vi "TestVirtual6.vi"(0 "reference in":refnum<class "G#SubSubClass1.lvclass">, 5 "error in (no error)":errorcluster) -> (14 "reference out":refnum<class "G#SubSubClass1.lvclass">, 15 "MethodName":string[](array[string]), 19 "error out":errorcluster)   [LabVIEW 2010, in "G#SubSubClass1.lvclass"]
uses:
  G#SubSubClass1.lvclass
  G#SubClass1_class/G#SubClass1.lvclass
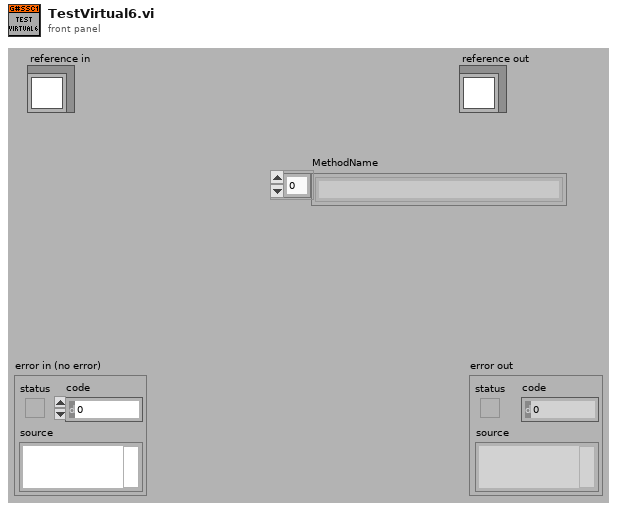
[diagram p1: front panel]
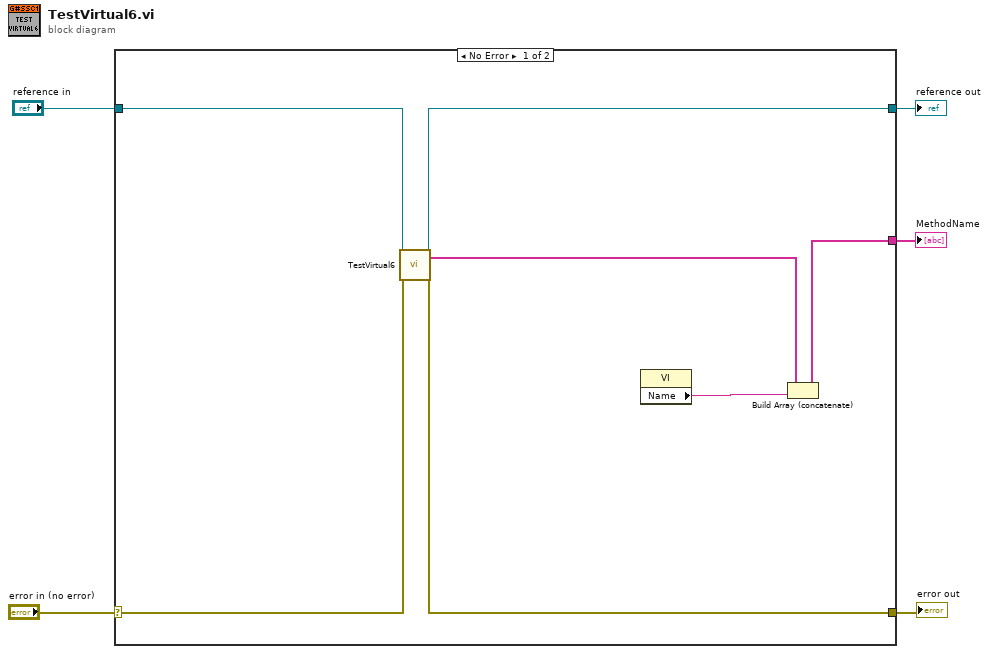
[diagram p0: block diagram]
diagram:
  n1 = case shown="No Error" "error in (no error)" {
    selector: "error in (no error)" -> [w10 w14]
    tunnel: [w9 w14] -> w4
    tunnel: [w11 w13] -> w2
    tunnel: "reference in" -> [w12 w13]
    tunnel: [w6 _] -> w1
    frame No Error {
      n2 = call-parent "TestVirtual6.vi"("reference in"=w12, "error in (no error)"=w10) -> ("reference out"=w11:refnum<class "G#SubSubClass1.lvclass">, "MethodName"=w7:string[], "error out"=w9:errorcluster)  [unwired: 15 in]
      n3 = property class="VI"() -> ("Name"=w8:string)  [unwired: 2 in, 2 out]
      n4 = Build Array (concatenate)(w7, w8) -> (w6:string[])
    }
    frame Error {
    }
  }
  "error out" <- w4
  "reference out" <- w2
  "MethodName" <- w1
